vi "Read timeout.vi"(8 "error in (no error)":errorcluster, 11 "Serial Data Unit in":refnum<class "Serial Data Unit.lvclass">) -> (0 "error out":errorcluster, 2 "timeout":u32=2000, 3 "Serial Data Unit out":refnum<class "Serial Data Unit.lvclass">)   [LabVIEW 2021, in "Serial Data Unit.lvclass"]
uses:
  Serial Data Unit.lvclass
  Serial Data Unit.lvclass/Serial Data Unit.ctl
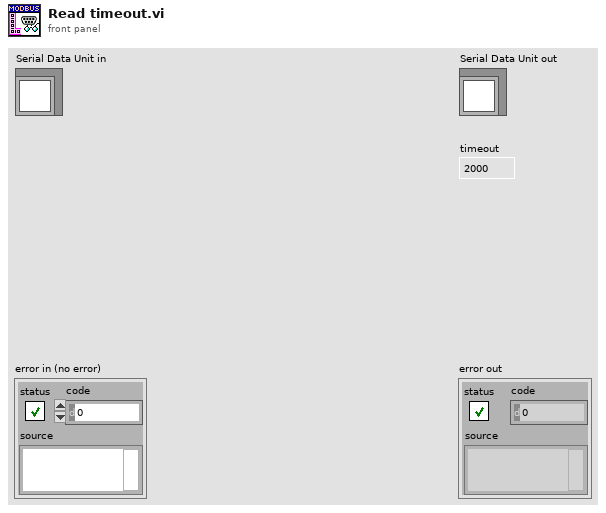
[diagram p1: front panel]
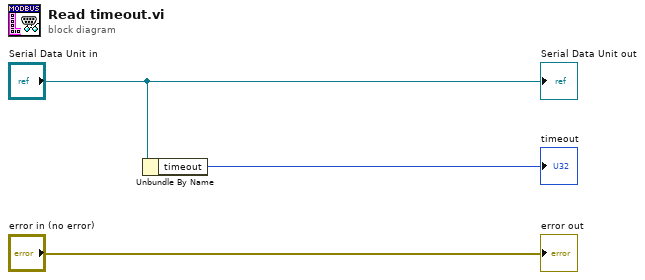
[diagram p0: block diagram]
diagram:
  n1 = Unbundle By Name("Serial Data Unit in") -> ("timeout"=→"timeout":u32)
  "error out" <- "error in (no error)"
  "Serial Data Unit out" <- "Serial Data Unit in"
